vi "get_config_cluster.vi"(8 "error in (no error)":errorcluster, 11 "StimulatorDL090503 in":refnum<class "StimulatorDL090503.lvclass">) -> (0 "error out":errorcluster, 2 "config cluster (variant)":variant, 3 "StimulatorDL090503 out":refnum<class "StimulatorDL090503.lvclass">)   [LabVIEW 2010, in "StimulatorDL090503.lvclass"]
uses:
  StimulatorDL090503.lvclass
  StimulatorDL090503.lvclass/StimulatorDL090503.ctl
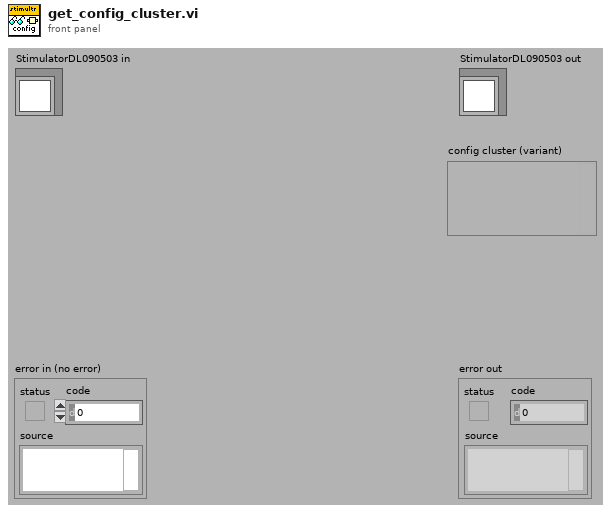
[diagram p1: front panel]
types:
  T1 = typedef "StimulatorDL090503.lvclass/config_data_cluster.ctl" = cluster{"signalWriter":T2, "sampling rate":dbl[unit]}
  T2 = typedef "plugin_specification.ctl" = cluster{"class path":string, "configuration":string, "label":string, "settings name":string}
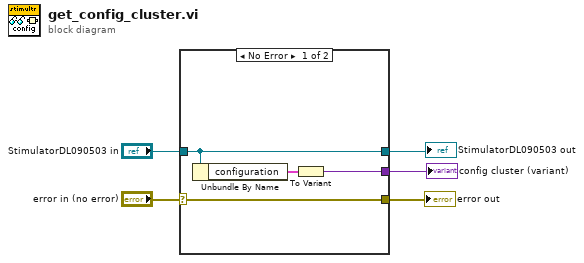
[diagram p0: block diagram]
diagram:
  n1 = case shown="No Error" "error in (no error)" {
    selector: "error in (no error)" -> [w7 w10]
    tunnel: "StimulatorDL090503 in" -> [w6 w11]
    tunnel: [w8 _] -> w3
    tunnel: [w7 w10] -> w2
    tunnel: [w6 w11] -> w1
    frame No Error {
      n2 = Unbundle By Name(w6) -> ("configuration"=w9:T1)
      n3 = To Variant(anything=w9) -> (Variant=w8:variant)
    }
    frame Error {
    }
  }
  "error out" <- w2
  "StimulatorDL090503 out" <- w1
  "config cluster (variant)" <- w3
